vi "Parse Config File.vi"(8 "error in (no error)":errorcluster, 10 "Section":string, 11 "Config Path":path) -> (0 "error out":errorcluster, 3 "Array":T1[](array[typedef]))   [LabVIEW 2022 SP3, in "Read Configs Sections.lvlib"]
uses:
  Read Configs Sections.lvlib
  Section Data.ctl
  <vilib>/Utility/config.llb/Read Key (String).vi
  <vilib>/Utility/config.llb/Read Key (Path).vi
  <vilib>/Utility/config.llb/NI_LVConfig.lvlib
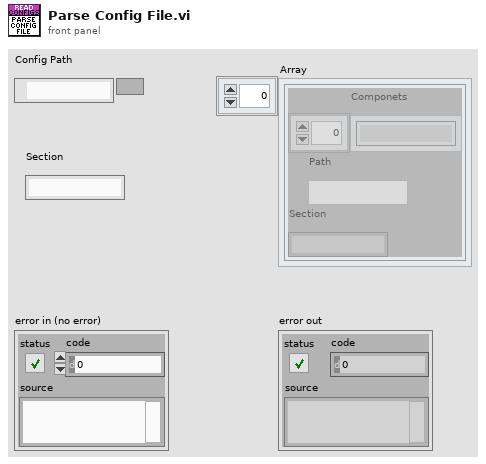
[diagram p1: front panel]
types:
  T1 = typedef "Read Configs Sections.lvlib/Section Data.ctl" = cluster{"Componets":string[], "Path":path, "Section":string}
  T2 = typedef "NI_LVConfig.lvlib/Config Data RefNum.ctl" = refnum<k1>
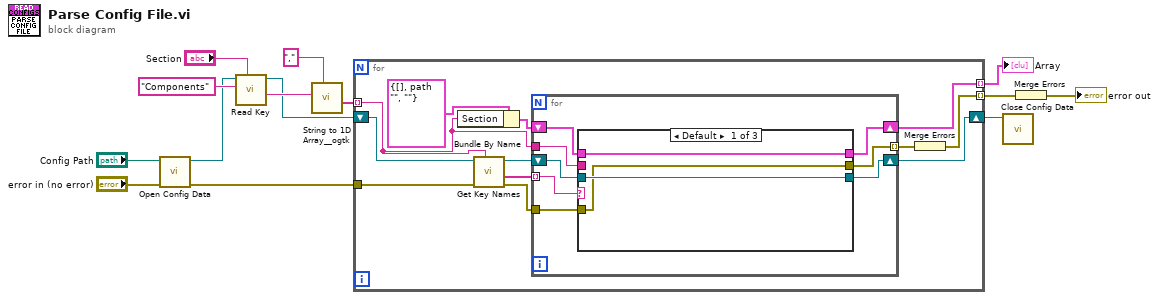
[diagram p0: block diagram]
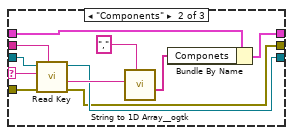
[diagram p2: hidden frame]
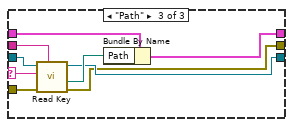
[diagram p3: hidden frame]
diagram:
  n1 = call <vilib>:"Open Config Data.vi"("error in (no error)"="error in (no error)", "configuration file path"="Config Path") -> ("error out"=w7:errorcluster, "refnum"=w3:T2)  [unwired: 7 in, 1 out]
  n2 = call-poly <vilib>:"Read Key.vi"("section"="Section", "key"="Components", "refnum"=w3) -> ("value"=w5:string, "refnum out"=w2:T2)  [unwired: 5 in, 2 out]
  n3 = call <userlib>:"String to 1D Array__ogtk.vi"("delimiter (Tab)"=",", "string"=w5) -> ("Array of Strings"=w4:string[])  [unwired: 9 in]
  n4 = for {
    tunnel: [w23] -> w13 mode=indexing
    shift-right: [w21] -> w1
    shift-left: w2 -> [w26]
    tunnel: w7 -> [w19]
    tunnel: [w16] -> w10 mode=indexing
    tunnel: w4 -> [w15] mode=indexing
    n5 = Bundle By Name(cluster=T1 {"Componets"=[], "Path"=path "", "Section"=""} ("Cluster"), "Section"=w15) -> (w22:T1)
    n6 = call <vilib>:"Get Key Names.vi"("section"=w15, "error in (no error)"=w19, "refnum"=w26) -> ("error out"=w18:errorcluster, "key names"=w25:string[], "refnum out"=w24:T2)  [unwired: 5 in, 1 out]
    n7 = for {
      tunnel: w25 -> [w31] mode=indexing
      tunnel: w15 -> [w30]
      shift-right: [w33] -> w23
      shift-left: w22 -> [w32]
      shift-right: [w29] -> w21
      shift-left: w24 -> [w34]
      tunnel: w18 -> [w28]
      tunnel: [w27] -> w17 mode=indexing
      n8 = case shown="Default" w31 {
        selector: w31 -> [_ w47 w56]
        tunnel: w34 -> [w36 w48 w57]
        tunnel: [w37 w46 w51] -> w33
        tunnel: w32 -> [w37 w45 w54]
        tunnel: w30 -> [_ w40 w55]
        tunnel: [w36 w41 w52] -> w29
        tunnel: w28 -> [w35 w39 w50]
        tunnel: [w35 w38 w49] -> w27
        frame Default {
        }
        frame "Components" {
          n9 = call-poly <vilib>:"Read Key.vi"("section"=w40, "error in (no error)"=w39, "key"=w47, "refnum"=w48) -> ("error out"=w38:errorcluster, "value"=w44:string, "refnum out"=w41:T2)  [unwired: 4 in, 1 out]
          n10 = call <userlib>:"String to 1D Array__ogtk.vi"("delimiter (Tab)"=",", "string"=w44) -> ("Array of Strings"=w43:string[])  [unwired: 9 in]
          n11 = Bundle By Name(cluster=w45, "Componets"=w43) -> (w46:T1)
        }
        frame "Path" {
          n12 = call-poly <vilib>:"Read Key.vi"("section"=w55, "error in (no error)"=w50, "key"=w56, "refnum"=w57) -> ("error out"=w49:errorcluster, "value"=w53:path, "refnum out"=w52:T2)  [unwired: 4 in, 1 out]
          n13 = Bundle By Name(cluster=w54, "Path"=w53) -> (w51:T1)
        }
      }
    }
    n14 = Merge Errors(w17) -> (w16:errorcluster)
  }
  "Array" <- w13
  n15 = call <vilib>:"Close Config Data.vi"("refnum"=w1) -> ()  [unwired: 9 in, 2 out]
  n16 = Merge Errors(w10) -> (→"error out":errorcluster)
